vi "LogStringTest.vi"() -> ()   [LabVIEW 2014]
uses:
  <vilib>/Rock Robotics/WPI/SerialPort/WPI_SerialPort.ctl
panel:
  in  "width (for increment)":i16
  out "Printed Incremental Value":i32
  in  "Increment":bool
  in  "File Name Set Before Running":string
  in  "SpecialTest":bool
  in  "Baud Rate":u32=460800
  in  "milliseconds to wait":u32=50
  out "Boolean":bool
  in  "Log string":string="TestTestTest"
  in  "stop":bool
  out "error out":errorcluster
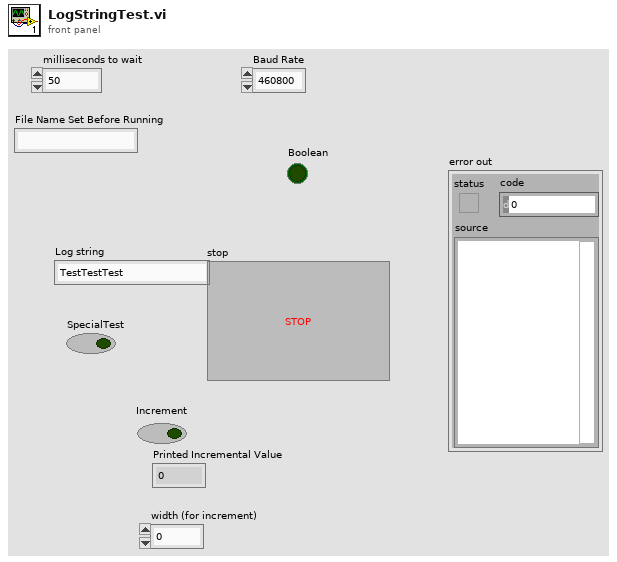
[diagram p1: front panel]
types:
  T1 = typedef "WPI_SerialPort.ctl" = enum16{"Onboard RS-232", "MXP TTL"}
  T2 = typedef "WPI_SerialPortRef.ctl" = cluster{"DevStatus":errorcluster, "Serial Port Name":refnum<visa-resource-name>}
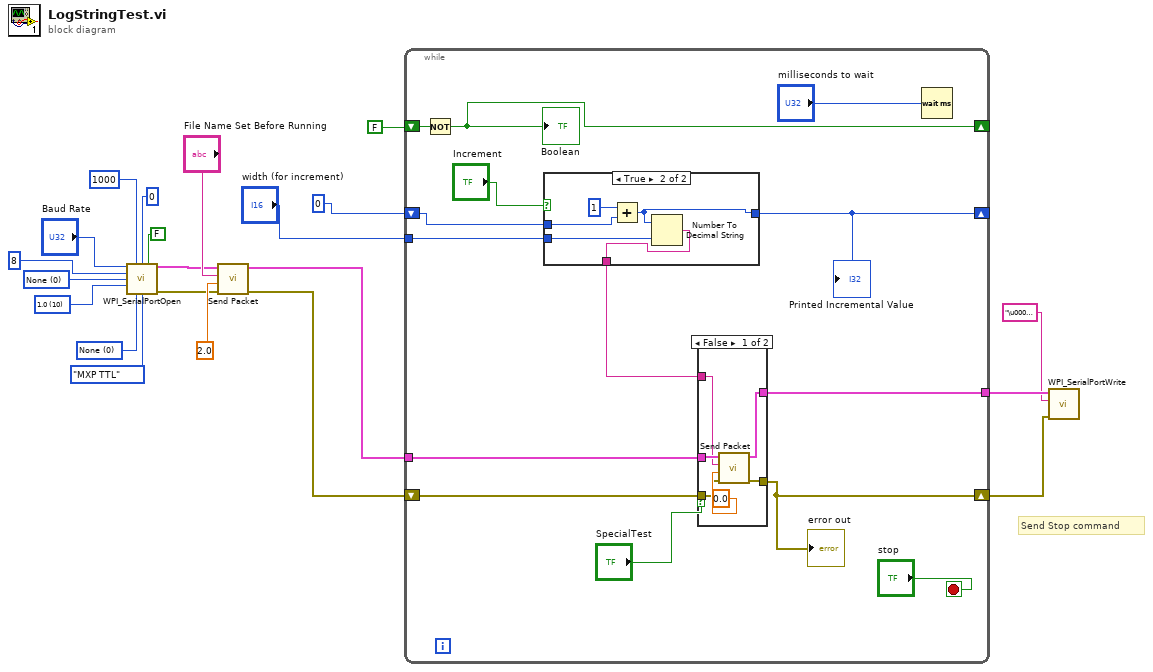
[diagram p0: block diagram]
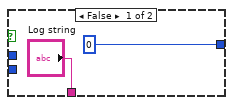
[diagram p2: hidden frame]
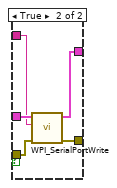
[diagram p3: hidden frame]
diagram:
  w15 = u16 10 items=["1.0"=10, "1.5"=15, "2.0"=20] ("Stop Bits")
  w16 = u16 0 items=["None", "Odd", "Even", "Mark", "Space"] ("Parity")
  w19 = u16 0 items=["None", "XON/XOFF", "RTS/CTS", "XON/XOFF & RTS/CTS", "DTR/DSR", "XON/XOFF & DTR/DSR"] ("Flow Control")
  # "Send Stop command"
  n1 = call <vilib>:"WPI_SerialPortOpen.vi"("Baud Rate"="Baud Rate", "Timeout Value (ms)"=u32 1000, "Termination Char (0xA = '\\n' = LF)"=u8 0 ("Termination Char (0xA = '\\n' = LF)"), "Enable Termination Char? (T)"=FALSE, "Data Bits"=u16 8, "Parity"=w16, "Stop Bits"=w15, "Flow Control"=w19, "Serial Port"=WPI_SerialPort."MXP TTL") -> ("SerialPortRef"=w7:T2, "error out"=w9:errorcluster)  [unwired: 5 in]
  n2 = call "Send Packet.vi"("error in (no error)"=w9, "Log Type"=2.0, "Log string"="File Name Set Before Running", "SerialPortRef"=w7) -> ("error out"=w8:errorcluster, "SerialPortRef out"=w6:T2)  [unwired: 4 in]
  n3 = while {
    tunnel: w6 -> [w30]
    shift-right: [w32] -> _
    shift-left: FALSE -> [w33]
    shift-right: [w28] -> w2
    shift-left: w8 -> [w31]
    shift-right: [w26] -> _
    shift-left: 0 -> [w25]
    tunnel: "width (for increment)" -> [w23]
    tunnel: [w22] -> w3
    stop <- "stop" stop-if-true
    n4 = Not(x=w33) -> (.not. x?=w32:bool)
    "Boolean" <- w32
    n5 = case shown="True" "Increment" {
      tunnel: [0 w40] -> w26
      tunnel: w25 -> [_ w42]
      tunnel: ["Log string" w39] -> w24
      tunnel: w23 -> [_ w38]
      frame False {
      }
      frame True {
        n6 = Add(x=1, y=w42) -> (x+y=w40:i32)
        n7 = Number To Decimal String(number=w40, width (-)=w38) -> (decimal integer string=w39:string)
      }
    }
    "Printed Incremental Value" <- w26
    n8 = case shown="False" "SpecialTest" {
      tunnel: [w46 w53] -> w28
      tunnel: w31 -> [w47 w52]
      tunnel: w30 -> [w45 w51]
      tunnel: w24 -> [w44 w50]
      tunnel: [w43 w49] -> w22
      frame False {
        n9 = call "Send Packet.vi"("error in (no error)"=w47, "Log Type"=0.0, "Log string"=w44, "SerialPortRef"=w45) -> ("error out"=w46:errorcluster, "SerialPortRef out"=w43:T2)  [unwired: 4 in]
      }
      frame True {
        n10 = call <vilib>:"WPI_SerialPortWrite.vi"("error in (no error)"=w52, "Buffer"=w50, "SerialPortRef"=w51) -> ("error out"=w53:errorcluster, "SerialPortRef"=w49:T2)  [unwired: 6 in, 1 out]
      }
    }
    "error out" <- w28
    n11 = Wait (ms)(milliseconds to wait="milliseconds to wait") -> ()  [unwired: 1 out]
  }
  n12 = call <vilib>:"WPI_SerialPortWrite.vi"("error in (no error)"=w2, "Buffer"="\u0004\u0004", "SerialPortRef"=w3) -> ()  [unwired: 6 in, 3 out]
